vi "Parse_Triangulated_file.vi"() -> ()   [LabVIEW 2011]
panel:
  in  "File Contains Both Faces?":bool
  in  "File Prefix":string="obj"
  out "norm":string
  out "vert":string
  out "string":string
  in  "File to Parse":path
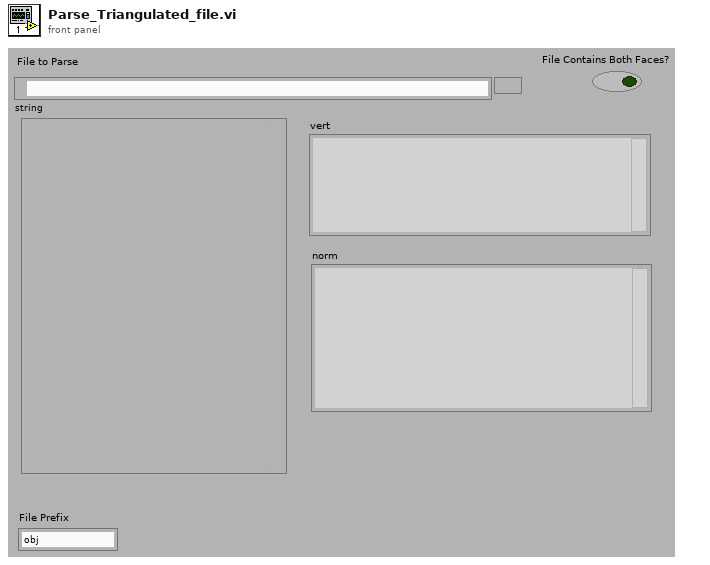
[diagram p1: front panel]
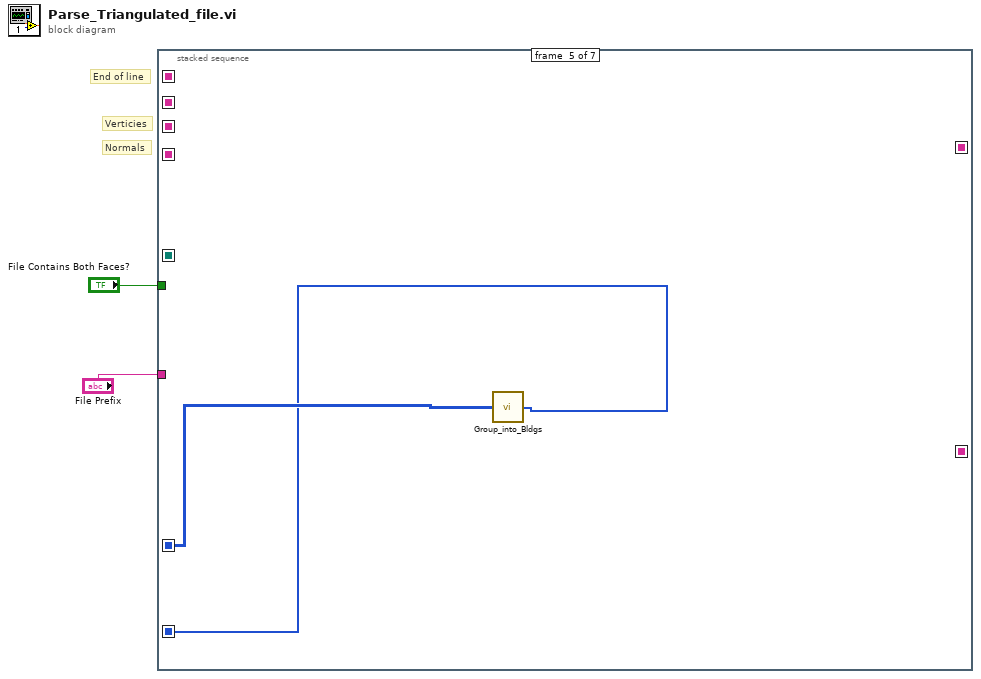
[diagram p0: block diagram]
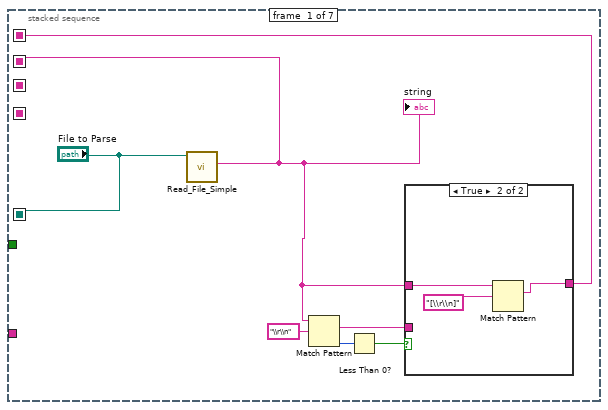
[diagram p2: hidden frame]
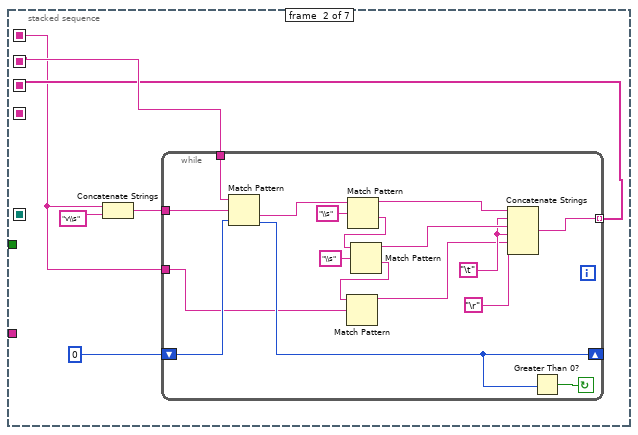
[diagram p4: hidden frame]
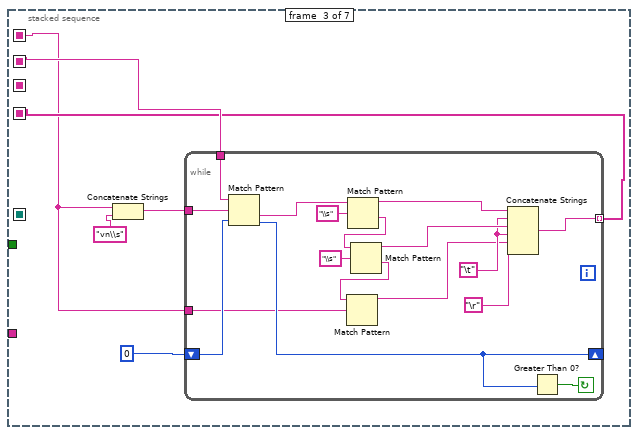
[diagram p5: hidden frame]
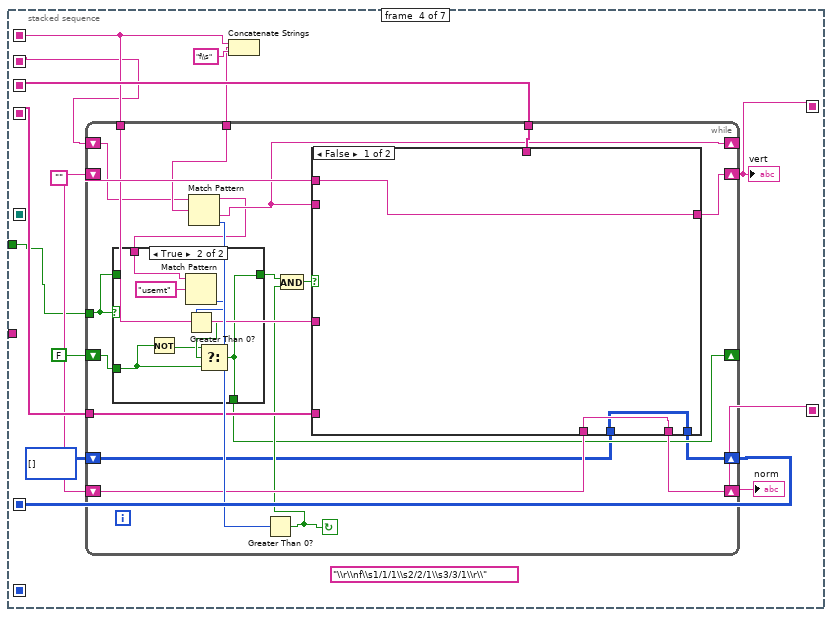
[diagram p6: hidden frame]
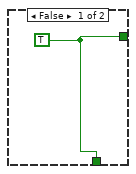
[diagram p7: hidden frame]
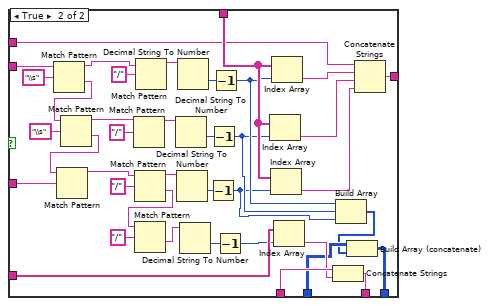
[diagram p8: hidden frame]
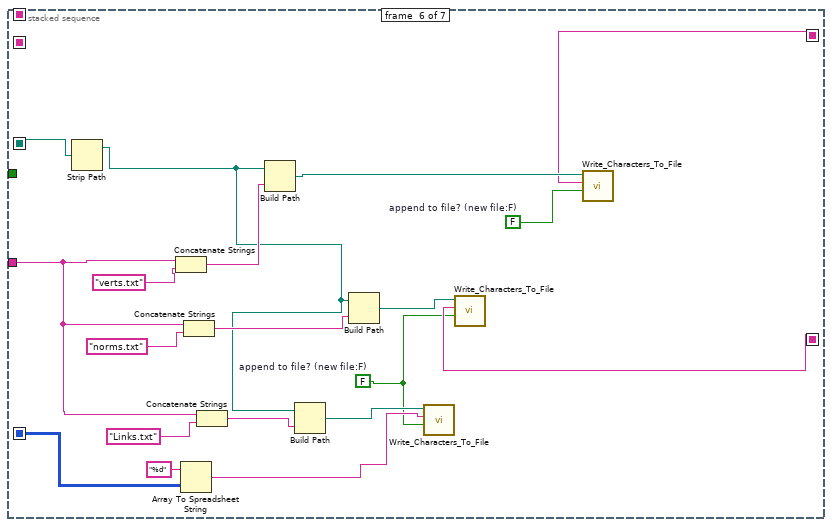
[diagram p9: hidden frame]
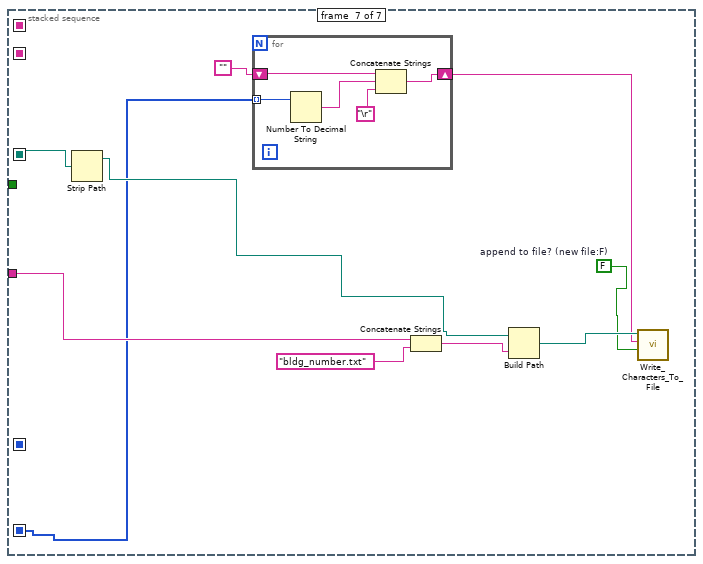
[diagram p10: hidden frame]
diagram:
  # "End of line"
  # "Normals"
  # "Verticies"
  n1 = stacked-sequence {
    seq-local: [w3 _ _ _ _ _ _] -> [_ w19 w42 w64 _ _ _]
    seq-local: [_ w17 _ _ _ _ _] -> [_ _ _ w72 _ _ _]
    seq-local: [_ _ w40 _ _ _ _] -> [_ _ _ w71 _ _ _]
    seq-local: [_ _ _ w69 _ _ _] -> [_ _ _ _ _ w160 _]
    seq-local: [_ _ _ w68 _ _ _] -> [_ _ _ _ _ w155 _]
    seq-local: ["File to Parse" _ _ _ _ _ _] -> [_ _ _ _ _ w163 w173]
    seq-local: [w5 _ _ _ _ _ _] -> [_ w15 w37 w66 _ _ _]
    seq-local: [_ _ _ w60 _ _ _] -> [_ _ _ _ w144 w153 _]
    seq-local: [_ _ _ _ w143 _ _] -> [_ _ _ _ _ _ w165]
    tunnel: "File Prefix" -> [_ _ _ _ _ w145 w167]
    tunnel: "File Contains Both Faces?" -> [_ _ _ w62 _ _ _]
    frame #0 {
      n2 = call "Read_File_Simple.vi"("Filename"="File to Parse") -> ("string"=w3:string)  [unwired: 4 in, 5 out]
      "string" <- w3
      n3 = Match Pattern(string=w3, regular expression="\\r\\n") -> (match substring=w4:string, offset past match=w8:i32)  [unwired: 1 in, 2 out]
      n4 = Less Than 0?(x=w8) -> (x < 0?=w7:bool)
      n5 = case shown="True" w7 {
        tunnel: w3 -> [_ w13]
        tunnel: [w10 w11] -> w5
        tunnel: w4 -> [w10 _]
        frame False {
        }
        frame True {
          n6 = Match Pattern(string=w13, regular expression="[\\r\\n]") -> (match substring=w11:string)  [unwired: 1 in, 3 out]
        }
      }
    }
    frame #1 {
      n7 = Concatenate Strings(w15, "v\\s" ("regular expression")) -> (w14:string)
      n8 = while {
        tunnel: w19 -> [w36]
        shift-right: [w28] -> _
        shift-left: 0 ("offset past match") -> [w35]
        tunnel: [w29] -> w17 mode=indexing
        tunnel: w15 -> [w21]
        tunnel: w14 -> [w20]
        stop <- w27 continue-if-true
        w24 = "\t"
        n9 = Match Pattern(string=w36, regular expression=w20, offset (0)=w35) -> (after substring=w33:string, offset past match=w28:i32)  [unwired: 2 out]
        n10 = Match Pattern(string=w33, regular expression="\\s") -> (before substring=w26:string, after substring=w31:string)  [unwired: 1 in, 2 out]
        n11 = Match Pattern(string=w31, regular expression="\\s") -> (before substring=w25:string, after substring=w30:string)  [unwired: 1 in, 2 out]
        n12 = Match Pattern(string=w30, regular expression=w21) -> (before substring=w23:string)  [unwired: 1 in, 3 out]
        n13 = Concatenate Strings(w26, w24, w25, w24, w23, "\r") -> (w29:string)
        n14 = Greater Than 0?(x=w28) -> (x > 0?=w27:bool)
      }
    }
    frame #2 {
      n15 = Concatenate Strings(w37, "vn\\s" ("regular expression")) -> (w38:string)
      n16 = while {
        tunnel: w42 -> [w59]
        shift-right: [w51] -> _
        shift-left: 0 ("offset past match") -> [w58]
        tunnel: [w52] -> w40 mode=indexing
        tunnel: w38 -> [w44]
        tunnel: w37 -> [w43]
        stop <- w50 continue-if-true
        w47 = "\t"
        n17 = Match Pattern(string=w59, regular expression=w44, offset (0)=w58) -> (after substring=w56:string, offset past match=w51:i32)  [unwired: 2 out]
        n18 = Match Pattern(string=w56, regular expression="\\s") -> (before substring=w49:string, after substring=w54:string)  [unwired: 1 in, 2 out]
        n19 = Match Pattern(string=w54, regular expression="\\s") -> (before substring=w48:string, after substring=w53:string)  [unwired: 1 in, 2 out]
        n20 = Match Pattern(string=w53, regular expression=w43) -> (before substring=w46:string)  [unwired: 1 in, 3 out]
        n21 = Concatenate Strings(w49, w47, w48, w47, w46, "\r") -> (w52:string)
        n22 = Greater Than 0?(x=w51) -> (x > 0?=w50:bool)
      }
    }
    frame #3 {
      w70 = ""
      (unwired) "\\r\\nf\\s1/1/1\\s2/2/1\\s3/3/1\\r\\"
      n23 = Concatenate Strings(w66, "f\\s" ("regular expression")) -> (w65:string)
      n24 = while {
        tunnel: w72 -> [w91]
        shift-right: [w89] -> w69
        shift-left: w70 -> [w90]
        tunnel: w71 -> [w88]
        shift-right: [w86] -> w68
        shift-left: w70 -> [w87]
        tunnel: w66 -> [w85]
        tunnel: w65 -> [w84]
        shift-right: [w80] -> _
        shift-left: w64 -> [w83]
        tunnel: w62 -> [w78]
        shift-right: [w75] -> _
        shift-left: FALSE -> [w76]
        shift-right: [w73] -> w60
        shift-left: i32[][] [] -> [w74]
        stop <- w81 continue-if-true
        n25 = Match Pattern(string=w83, regular expression=w84) -> (before substring=w77:string, after substring=w80:string, offset past match=w92:i32)  [unwired: 1 in, 1 out]
        n26 = case shown="True" w78 {
          tunnel: [w93 w94] -> w79
          tunnel: w78 -> [_ _]
          tunnel: w77 -> [_ w98]
          tunnel: w76 -> [_ w95]
          tunnel: [w93 w94] -> w75
          frame False {
            w93 = TRUE
          }
          frame True {
            n27 = Not(x=w95) -> (.not. x?=w96:bool)
            n28 = Match Pattern(string=w98, regular expression="usemt") -> (offset past match=w99:i32)  [unwired: 1 in, 3 out]
            n29 = Greater Than 0?(x=w99) -> (x > 0?=w97:bool)
            n30 = Select(t=w96, s=w97, f=w95) -> (s? t:f=w94:bool)
          }
        }
        n31 = Greater Than 0?(x=w92) -> (x > 0?=w81:bool)
        n32 = And(x=w79, y=w81) -> (x .and. y?=w82:bool)
        n33 = case shown="False" w82 {
          tunnel: w80 -> [_ w141]
          tunnel: w91 -> [_ w126]
          tunnel: w90 -> [w103 w122]
          tunnel: [w103 w121] -> w89
          tunnel: w88 -> [_ w116]
          tunnel: w87 -> [w102 w115]
          tunnel: [w102 w113] -> w86
          tunnel: w85 -> [_ w110]
          tunnel: w74 -> [w101 w106]
          tunnel: [w101 w104] -> w73
          frame False {
          }
          frame True {
            n34 = Match Pattern(string=w141, regular expression="\\s") -> (before substring=w136:string, after substring=w139:string)  [unwired: 1 in, 2 out]
            n35 = Match Pattern(string=w139, regular expression="\\s") -> (before substring=w128:string, after substring=w138:string)  [unwired: 1 in, 2 out]
            n36 = Match Pattern(string=w138, regular expression=w110) -> (before substring=w127:string)  [unwired: 1 in, 3 out]
            n37 = Match Pattern(string=w128, regular expression="/") -> (before substring=w132:string)  [unwired: 1 in, 3 out]
            n38 = Match Pattern(string=w127, regular expression="/") -> (before substring=w119:string, after substring=w111:string)  [unwired: 1 in, 2 out]
            n39 = Match Pattern(string=w111, regular expression="/") -> (after substring=w117:string)  [unwired: 1 in, 3 out]
            n40 = Match Pattern(string=w136, regular expression="/") -> (before substring=w135:string)  [unwired: 1 in, 3 out]
            n41 = Decimal String To Number(string=w132) -> (number=w133:i32)  [unwired: 2 in, 1 out]
            n42 = Decimal String To Number(string=w119) -> (number=w129:i32)  [unwired: 2 in, 1 out]
            n43 = Decimal String To Number(string=w135) -> (number=w134:i32)  [unwired: 2 in, 1 out]
            n44 = Decimal String To Number(string=w117) -> (number=w118:i32)  [unwired: 2 in, 1 out]
            n45 = Decrement(x=w129) -> (x-1=w107:i32)
            n46 = Decrement(x=w133) -> (x-1=w108:i32)
            n47 = Decrement(x=w134) -> (x-1=w109:i32)
            n48 = Decrement(x=w118) -> (x-1=w112:i32)
            n49 = Index Array(array=w126, index=w108) -> (element=w124:string)
            n50 = Index Array(array=w126, index=w107) -> (element=w123:string)
            n51 = Index Array(array=w126, index=w109) -> (element=w125:string)
            n52 = Index Array(array=w116, index=w112) -> (element=w114:string)
            n53 = Concatenate Strings(w115, w114) -> (w113:string)
            n54 = Build Array(w109, w108, w107) -> (w105:i32[])
            n55 = Build Array (concatenate)(w106, w105) -> (w104:i32[][])
            n56 = Concatenate Strings(w122, w125, w124, w123) -> (w121:string)
          }
        }
      }
      "vert" <- w69
      "norm" <- w68
    }
    frame #4 {
      n57 = call "Group_into_Bldgs.vi"("Facet Verticies"=w144) -> ("Bldgs Number"=w143:i32[])  [unwired: 2 in]
    }
    frame #5 {
      w146 = FALSE  # append to file? (new file:F)
      w154 = FALSE  # append to file? (new file:F)
      n58 = Strip Path(path=w163) -> (stripped path=w147:path)  [unwired: 1 out]
      n59 = Concatenate Strings(w145, "verts.txt" ("string")) -> (w162:string)
      n60 = Array To Spreadsheet String(array=w153, 3:"%d" ("format string")) -> (spreadsheet string=w149:string)  [unwired: 1 in]
      n61 = Concatenate Strings(w145, "norms.txt" ("string")) -> (w157:string)
      n62 = Concatenate Strings(w145, "Links.txt" ("string")) -> (w151:string)
      n63 = Build Path(base path=w147, name or relative path=w162) -> (appended path=w161:path)
      n64 = Build Path(base path=w147, name or relative path=w151) -> (appended path=w150:path)
      n65 = Build Path(base path=w147, name or relative path=w157) -> (appended path=w156:path)
      n66 = call "Write_Characters_To_File.vi"("file path (dialog if empty)"=w150, "character string"=w149, "append to file? (new file:F)"=w146) -> ()  [unwired: 5 in, 1 out]
      n67 = call "Write_Characters_To_File.vi"("file path (dialog if empty)"=w156, "character string"=w155, "append to file? (new file:F)"=w146) -> ()  [unwired: 5 in, 1 out]
      n68 = call "Write_Characters_To_File.vi"("file path (dialog if empty)"=w161, "character string"=w160, "append to file? (new file:F)"=w154) -> ()  [unwired: 5 in, 1 out]
    }
    frame #6 {
      w168 = FALSE  # append to file? (new file:F)
      n69 = Strip Path(path=w173) -> (stripped path=w169:path)  [unwired: 1 out]
      n70 = for {
        shift-right: [w174] -> w164
        shift-left: "" -> [w178]
        tunnel: w165 -> [w177] mode=indexing
        n71 = Number To Decimal String(number=w177) -> (decimal integer string=w176:string)  [unwired: 1 in]
        n72 = Concatenate Strings(w178, w176, "\r") -> (w174:string)
      }
      n73 = Concatenate Strings(w167, "bldg_number.txt" ("string")) -> (w171:string)
      n74 = Build Path(base path=w169, name or relative path=w171) -> (appended path=w172:path)
      n75 = call "Write_Characters_To_File.vi"("file path (dialog if empty)"=w172, "character string"=w164, "append to file? (new file:F)"=w168) -> ()  [unwired: 5 in, 1 out]
    }
  }
